vi "2channel_mode.vi"() -> ()   [LabVIEW 2019]
panel:
  out "temperature":dynamicdata(graph)
  out "voltage":dynamicdata(graph)
  in  "stop (F)":bool
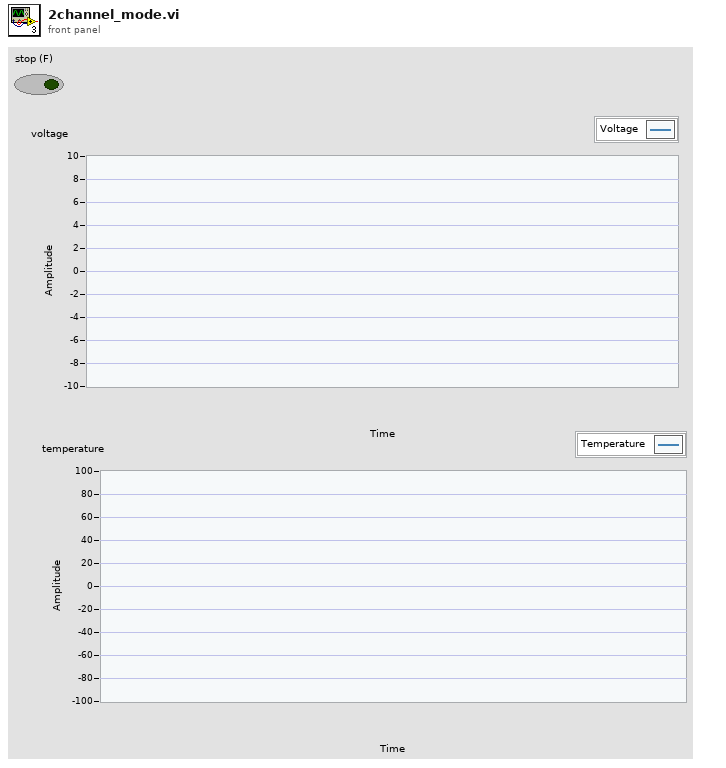
[diagram p1: front panel]
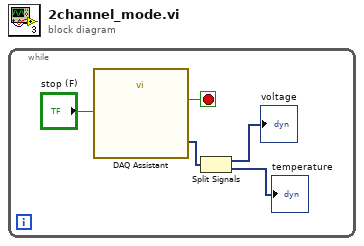
[diagram p0: block diagram]
diagram:
  n1 = while {
    stop <- w4 stop-if-true
    n2 = call "DAQ Assistant"("stop (F)"="stop (F)") -> ("data"=w3:dynamicdata, "stopped"=w4:bool)  [unwired: 15 in, 2 out]
    n3 = Split Signals(w3) -> (→"voltage":dynamicdata, →"temperature":dynamicdata)  [unwired: 2 in]
  }
